vi "Current_Linear_Speed.vi"(10 "Linear Distance prev":dbl, 11 "Linear Distance":dbl) -> (2 "Change In Linear Distance":dbl, 3 "Current Linear Speed":dbl)   [LabVIEW 2018]
doc: "This VI calculates the change in linear distance by subtracting previous linear distance from current linear distance. It also calculates current linear speed by dividing change in linear distance by change in time (0.1 s).\n\nInputs:\nLinear distance prev;\nLinear distance.\n\nOutputs:\nCurrent Linear speed;\nChange in linear distance."
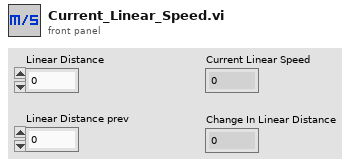
[diagram p1: front panel]
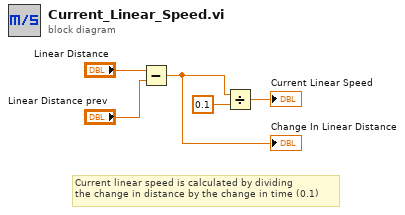
[diagram p0: block diagram]
diagram:
  # "Current linear speed is calculated by dividing \nthe change in distance by the change in time (0.1)"
  n1 = Subtract(x="Linear Distance", y="Linear Distance prev") -> (x-y=w1:dbl)
  "Change In Linear Distance" <- w1
  n2 = Divide(x=w1, y=0.1) -> (x/y=→"Current Linear Speed":dbl)
